vi "WebView2 Viewer.vi"(2 "ProjectRef":refnum<vi>, 4 "Extra Scripts":string, 5 "FileDependency In":map{path, T1}(c390), 6 "Options":string, 7 "OpenWebBrowser(False)":bool, 8 "error in":errorcluster, 9 "Embedd VISJS Librarya in HTMl File(False)":bool, 10 "HTMLFilePath":path, 11 "LibraryDependency":map{path, T3}(c390)) -> (0 "error out":errorcluster, 3 "HTMLFileContent":string)   [LabVIEW 2020, in "WebView2-Viewer.lvlib"] (continued)
if(d)e=g.iterator;else if(h)e=g;else{if(!(C=Wy(g)))throw new Uy(Gy(g)+\" is not iterable\");if(jy(C)){for(I=0,i=Ly(g);i>I;I++)if((o=p(g[I]))&&Vy(Ky,o))return o;return new _y(!1)}e=Yy(g,C)}for(n=d?g.next:e.next;!(r=Zy(n,e)).done;){try{o=p(r.value)}catch(g){Qy(e,\"throw\",g)}if(\"object\"==typeof o&&o&&Vy(Ky,o))return o}return new _y(!1)},Xy=og,Jy=TypeError,qy=function(g,t){if(Xy(t,g))return g;throw new Jy(\"Incorrect invocation\")},$y=TA,gm=C,tm=zy,Am=I,em=uA,Cm=Hy,Im=qy,im=O,om=gg,nm=Q,rm=_I,sm=Jt.f,am=Sr.forEach,dm=D,hm=GC.set,lm=GC.getterFor,cm=function(g,t,A){var e,C=-1!==g.indexOf(\"Map\"),I=-1!==g.indexOf(\"Weak\"),i=C?\"set\":\"add\",o=gm[g],n=o&&o.prototype,r={};if(dm&&im(o)&&(I||n.forEach&&!Am((function(){(new o).entries().next()})))){var s=(e=t((function(t,A){hm(Im(t,s),{type:g,collection:new o}),nm(A)||Cm(A,t[i],{that:t,AS_ENTRIES:C})}))).prototype,a=lm(g);am([\"add\",\"clear\",\"delete\",\"forEach\",\"get\",\"has\",\"set\",\"keys\",\"values\",\"entries\"],(function(g){var t=\"add\"===g||\"set\"===g;!(g in n)||I&&\"clear\"===g||em(s,g,(function(A,e){var C=a(this).collection;if(!t&&I&&!om(A))return\"get\"===g&&void 0;var i=C[g](0===A?0:A,e);return t?this:i}))})),I||sm(s,\"size\",{configurable:!0,get:function(){return a(this).collection.size}})}else e=A.getConstructor(t,g,C,i),tm.enable();return rm(e,g,!1,!0),r[g]=e,$y({global:!0,forced:!0},r),I||A.setStrong(e,g,C),e},um=TI,pm=function(g,t,A){for(var e in t)A&&A.unsafe&&g[e]?g[e]=t[e]:um(g,e,t[e],A);return g},fm=ig,vm=ur,ym=D,mm=dt(\"species\"),bm=function(g){var t=fm(g);ym&&t&&!t[mm]&&vm(t,mm,{configurable:!0,get:function(){return this}})},wm=pI,km=ur,xm=pm,Em=Xt,Om=qy,Tm=Q,Dm=Hy,Nm=Ei,Rm=Oi,Pm=bm,Mm=D,Bm=zy.fastKey,zm=GC.set,Sm=GC.getterFor,Zm={getConstructor:function(g,t,A,e){var C=g((function(g,C){Om(g,I),zm(g,{type:t,index:wm(null),first:void 0,last:void 0,size:0}),Mm||(g.size=0),Tm(C)||Dm(C,g[e],{that:g,AS_ENTRIES:A})})),I=C.prototype,i=Sm(t),o=function(g,t,A){var e,C,I=i(g),o=n(g,t);return o?o.value=A:(I.last=o={index:C=Bm(t,!0),key:t,value:A,previous:e=I.last,next:void 0,removed:!1},I.first||(I.first=o),e&&(e.next=o),Mm?I.size++:g.size++,\"F\"!==C&&(I.index[C]=o)),g},n=function(g,t){var A,e=i(g),C=Bm(t);if(\"F\"!==C)return e.index[C];for(A=e.first;A;A=A.next)if(A.key===t)return A};return xm(I,{clear:function(){for(var g=i(this),t=g.index,A=g.first;A;)A.removed=!0,A.previous&&(A.previous=A.previous.next=void 0),delete t[A.index],A=A.next;g.first=g.last=void 0,Mm?g.size=0:this.size=0},delete:function(g){var t=this,A=i(t),e=n(t,g);if(e){var C=e.next,I=e.previous;delete A.index[e.index],e.removed=!0,I&&(I.next=C),C&&(C.previous=I),A.first===e&&(A.first=C),A.last===e&&(A.last=I),Mm?A.size--:t.size--}return!!e},forEach:function(g){for(var t,A=i(this),e=Em(g,arguments.length>1?arguments[1]:void 0);t=t?t.next:A.first;)for(e(t.value,t.key,this);t&&t.removed;)t=t.previous},has:function(g){return!!n(this,g)}}),xm(I,A?{get:function(g){var t=n(this,g);return t&&t.value},set:function(g,t){return o(this,0===g?0:g,t)}}:{add:function(g){return o(this,g=0===g?0:g,g)}}),Mm&&km(I,\"size\",{configurable:!0,get:function(){return i(this).size}}),C},setStrong:function(g,t,A){var e=t+\" Iterator\",C=Sm(t),I=Sm(e);Nm(g,t,(function(g,t){zm(this,{type:e,target:g,state:C(g),kind:t,last:void 0})}),(function(){for(var g=I(this),t=g.kind,A=g.last;A&&A.removed;)A=A.previous;return g.target&&(g.last=A=A?A.next:g.state.first)?Rm(\"keys\"===t?A.key:\"values\"===t?A.value:[A.key,A.value],!1):(g.target=void 0,Rm(void 0,!0))}),A?\"entries\":\"values\",!A,!0),Pm(t)}};cm(\"Map\",(function(g){return function(){return g(this,arguments.length?arguments[0]:void 0)}}),Zm);var Fm=A(tg.Map),Gm=function(){function g(){cn(this,g),this.clear(),this._defaultIndex=0,this._groupIndex=0,this._defaultGroups=[{border:\"#2B7CE9\",background:\"#97C2FC\",highlight:{border:\"#2B7CE9\",background:\"#D2E5FF\"},hover:{border:\"#2B7CE9\",background:\"#D2E5FF\"}},{border:\"#FFA500\",background:\"#FFFF00\",highlight:{border:\"#FFA500\",background:\"#FFFFA3\"},hover:{border:\"#FFA500\",background:\"#FFFFA3\"}},{border:\"#FA0A10\",background:\"#FB7E81\",highlight:{border:\"#FA0A10\",background:\"#FFAFB1\"},hover:{border:\"#FA0A10\",background:\"#FFAFB1\"}},{border:\"#41A906\",background:\"#7BE141\",highlight:{border:\"#41A906\",background:\"#A1EC76\"},hover:{border:\"#41A906\",background:\"#A1EC76\"}},{border:\"#E129F0\",background:\"#EB7DF4\",highlight:{border:\"#E129F0\",background:\"#F0B3F5\"},hover:{border:\"#E129F0\",background:\"#F0B3F5\"}},{border:\"#7C29F0\",background:\"#AD85E4\",highlight:{border:\"#7C29F0\",background:\"#D3BDF0\"},hover:{border:\"#7C29F0\",background:\"#D3BDF0\"}},{border:\"#C37F00\",background:\"#FFA807\",highlight:{border:\"#C37F00\",background:\"#FFCA66\"},hover:{border:\"#C37F00\",background:\"#FFCA66\"}},{border:\"#4220FB\",background:\"#6E6EFD\",highlight:{border:\"#4220FB\",background:\"#9B9BFD\"},hover:{border:\"#4220FB\",background:\"#9B9BFD\"}},{border:\"#FD5A77\",background:\"#FFC0CB\",highlight:{border:\"#FD5A77\",background:\"#FFD1D9\"},hover:{border:\"#FD5A77\",background:\"#FFD1D9\"}},{border:\"#4AD63A\",background:\"#C2FABC\",highlight:{border:\"#4AD63A\",background:\"#E6FFE3\"},hover:{border:\"#4AD63A\",background:\"#E6FFE3\"}},{border:\"#990000\",background:\"#EE0000\",highlight:{border:\"#BB0000\",background:\"#FF3333\"},hover:{border:\"#BB0000\",background:\"#FF3333\"}},{border:\"#FF6000\",background:\"#FF6000\",highlight:{border:\"#FF6000\",background:\"#FF6000\"},hover:{border:\"#FF6000\",background:\"#FF6000\"}},{border:\"#97C2FC\",background:\"#2B7CE9\",highlight:{border:\"#D2E5FF\",background:\"#2B7CE9\"},hover:{border:\"#D2E5FF\",background:\"#2B7CE9\"}},{border:\"#399605\",background:\"#255C03\",highlight:{border:\"#399605\",background:\"#255C03\"},hover:{border:\"#399605\",background:\"#255C03\"}},{border:\"#B70054\",background:\"#FF007E\",highlight:{border:\"#B70054\",background:\"#FF007E\"},hover:{border:\"#B70054\",background:\"#FF007E\"}},{border:\"#AD85E4\",background:\"#7C29F0\",highlight:{border:\"#D3BDF0\",background:\"#7C29F0\"},hover:{border:\"#D3BDF0\",background:\"#7C29F0\"}},{border:\"#4557FA\",background:\"#000EA1\",highlight:{border:\"#6E6EFD\",background:\"#000EA1\"},hover:{border:\"#6E6EFD\",background:\"#000EA1\"}},{border:\"#FFC0CB\",background:\"#FD5A77\",highlight:{border:\"#FFD1D9\",background:\"#FD5A77\"},hover:{border:\"#FFD1D9\",background:\"#FD5A77\"}},{border:\"#C2FABC\",background:\"#74D66A\",highlight:{border:\"#E6FFE3\",background:\"#74D66A\"},hover:{border:\"#E6FFE3\",background:\"#74D66A\"}},{border:\"#EE0000\",background:\"#990000\",highlight:{border:\"#FF3333\",background:\"#BB0000\"},hover:{border:\"#FF3333\",background:\"#BB0000\"}}],this.options={},this.defaultOptions={useDefaultGroups:!0},fe(this.options,this.defaultOptions)}return kd(g,[{key:\"setOptions\",value:function(g){var t=[\"useDefaultGroups\"];if(void 0!==g)for(var A in g)if(Object.prototype.hasOwnProperty.call(g,A)&&-1===Xc(t).call(t,A)){var e=g[A];this.add(A,e)}}},{key:\"clear\",value:function(){this._groups=new Fm,this._groupNames=[]}},{key:\"get\",value:function(g){var t=!(arguments.length>1&&void 0!==arguments[1])||arguments[1],A=this._groups.get(g);if(void 0===A&&t)if(!1===this.options.useDefaultGroups&&this._groupNames.length>0){var e=this._groupIndex%this._groupNames.length;++this._groupIndex,(A={}).color=this._groups.get(this._groupNames[e]),this._groups.set(g,A)}else{var C=this._defaultIndex%this._defaultGroups.length;this._defaultIndex++,(A={}).color=this._defaultGroups[C],this._groups.set(g,A)}return A}},{key:\"add\",value:function(g,t){return this._groups.has(g)||this._groupNames.push(g),this._groups.set(g,t),t}}]),g}();TA({target:\"Number\",stat:!0},{isNaN:function(g){return g!=g}});var jm=A(tg.Number.isNaN),Lm=C.isFinite,Vm=Number.isFinite||function(g){return\"number\"==typeof g&&Lm(g)};TA({target:\"Number\",stat:!0},{isFinite:Vm});var Ym=A(tg.Number.isFinite),Wm=Sr.some;TA({target:\"Array\",proto:!0,forced:!_h(\"some\")},{some:function(g){return Wm(this,g,arguments.length>1?arguments[1]:void 0)}});var Qm=Me(\"Array\").some,Um=og,_m=Qm,Km=Array.prototype,Hm=function(g){var t=g.some;return g===Km||Um(Km,g)&&t===Km.some?_m:t},Xm=A(Hm);function Jm(g){if(void 0===g)throw new ReferenceError(\"this hasn't been initialised - super() hasn't been called\");return g}var qm=qc,$m=A(qm);TA({target:\"Object\",stat:!0},{setPrototypeOf:ri});var gb=tg.Object.setPrototypeOf,tb=A(gb),Ab=A(Ge);function eb(g,t){var A;return eb=tb?Ab(A=tb).call(A):function(g,t){return g.__proto__=t,g},eb(g,t)}function Cb(g,t){if(\"function\"!=typeof t&&null!==t)throw new TypeError(\"Super expression must either be null or a function\");g.prototype=$m(t&&t.prototype,{constructor:{value:g,writable:!0,configurable:!0}}),kn(g,\"prototype\",{writable:!1}),t&&eb(g,t)}function Ib(g,t){if(t&&(\"object\"===yd(t)||\"function\"==typeof t))return t;if(void 0!==t)throw new TypeError(\"Derived constructors may only return object or undefined\");return Jm(g)}var ib=rc,ob=A(ib);function nb(g){var t;return nb=tb?Ab(t=ob).call(t):function(g){return g.__proto__||ob(g)},nb(g)}function rb(g,t,A){return(t=bd(t))in g?kn(g,t,{value:A,enumerable:!0,configurable:!0,writable:!0}):g[t]=A,g}var sb={exports:{}},ab={exports:{}};!function(g){var t=cd,A=fd;function e(C){return g.exports=e=\"function\"==typeof t&&\"symbol\"==typeof A?function(g){return typeof g}:function(g){return g&&\"function\"==typeof t&&g.constructor===t&&g!==t.prototype?\"symbol\":typeof g},g.exports.__esModule=!0,g.exports.default=g.exports,e(C)}g.exports=e,g.exports.__esModule=!0,g.exports.default=g.exports}(ab);var db=ab.exports,hb=el,lb=qg,cb=Dh,ub=T,pb=Jt,fb=gg,vb=uA,yb=Error,mb=u(\"\".replace),bb=String(new yb(\"zxcasd\").stack),wb=/\\n\\s*at [^:]*:[^\\n]*/,kb=wb.test(bb),xb=G,Eb=!I((function(){var g=new Error(\"a\");return!(\"stack\"in g)||(Object.defineProperty(g,\"stack\",xb(1,7)),7!==g.stack)})),Ob=uA,Tb=function(g,t){if(kb&&\"string\"==typeof g&&!yb.prepareStackTrace)for(;t--;)g=mb(g,wb,\"\");return g},Db=Eb,Nb=Error.captureStackTrace,Rb=sC,Pb=TA,Mb=og,Bb=EI,zb=ri,Sb=function(g,t,A){for(var e=cb(t),C=pb.f,I=ub.f,i=0;i<e.length;i++){var o=e[i];lb(g,o)||A&&lb(A,o)||C(g,o,I(t,o))}},Zb=pI,Fb=uA,Gb=G,jb=function(g,t){fb(t)&&\"cause\"in t&&vb(g,\"cause\",t.cause)},Lb=function(g,t,A,e){Db&&(Nb?Nb(g,t):Ob(g,\"stack\",Tb(A,e)))},Vb=Hy,Yb=function(g,t){return void 0===g?arguments.length<2?\"\":t:Rb(g)},Wb=dt(\"toStringTag\"),Qb=Error,Ub=[].push,_b=function(g,t){var A,e=Mb(Kb,this);zb?A=zb(new Qb,e?Bb(this):Kb):(A=e?this:Zb(Kb),Fb(A,Wb,\"Error\")),void 0!==t&&Fb(A,\"message\",Yb(t)),Lb(A,_b,A.stack,1),arguments.length>2&&jb(A,arguments[2]);var C=[];return Vb(g,Ub,{that:C}),Fb(A,\"errors\",C),A};zb?zb(_b,Qb):Sb(_b,Qb,{name:!0});var Kb=_b.prototype=Zb(Qb.prototype,{constructor:Gb(1,_b),message:Gb(1,\"\"),name:Gb(1,\"AggregateError\")});Pb({global:!0,constructor:!0,arity:2},{AggregateError:_b});var Hb,Xb,Jb,qb,$b=\"process\"===y(C.process),gw=ro,tw=Og,Aw=TypeError,ew=function(g){if(gw(g))return g;throw new Aw(tw(g)+\" is not a constructor\")},Cw=AA,Iw=ew,iw=Q,ow=dt(\"species\"),nw=function(g,t){var A,e=Cw(g).constructor;return void 0===e||iw(A=Cw(e)[ow])?t:Iw(A)},rw=/(?:ipad|iphone|ipod).*applewebkit/i.test(ng),sw=C,aw=a,dw=Xt,hw=O,lw=qg,cw=I,uw=gI,pw=ve,fw=Et,vw=iu,yw=rw,mw=$b,bw=sw.setImmediate,ww=sw.clearImmediate,kw=sw.process,xw=sw.Dispatch,Ew=sw.Function,Ow=sw.MessageChannel,Tw=sw.String,Dw=0,Nw={},Rw=\"onreadystatechange\";cw((function(){Hb=sw.location}));var Pw=function(g){if(lw(Nw,g)){var t=Nw[g];delete Nw[g],t()}},Mw=function(g){return function(){Pw(g)}},Bw=function(g){Pw(g.data)},zw=function(g){sw.postMessage(Tw(g),Hb.protocol+\"//\"+Hb.host)};bw&&ww||(bw=function(g){vw(arguments.length,1);var t=hw(g)?g:Ew(g),A=pw(arguments,1);return Nw[++Dw]=function(){aw(t,void 0,A)},Xb(Dw),Dw},ww=function(g){delete Nw[g]},mw?Xb=function(g){kw.nextTick(Mw(g))}:xw&&xw.now?Xb=function(g){xw.now(Mw(g))}:Ow&&!yw?(qb=(Jb=new Ow).port2,Jb.port1.onmessage=Bw,Xb=dw(qb.postMessage,qb)):sw.addEventListener&&hw(sw.postMessage)&&!sw.importScripts&&Hb&&\"file:\"!==Hb.protocol&&!cw(zw)?(Xb=zw,sw.addEventListener(\"message\",Bw,!1)):Xb=Rw in fw(\"script\")?function(g){uw.appendChild(fw(\"script\"))[Rw]=function(){uw.removeChild(this),Pw(g)}}:function(g){setTimeout(Mw(g),0)});var Sw={set:bw,clear:ww},Zw=function(){this.head=null,this.tail=null};Zw.prototype={add:function(g){var t={item:g,next:null},A=this.tail;A?A.next=t:this.head=t,this.tail=t},get:function(){var g=this.head;if(g)return null===(this.head=g.next)&&(this.tail=null),g.item}};var Fw,Gw,jw,Lw,Vw,Yw=Zw,Ww=/ipad|iphone|ipod/i.test(ng)&&\"undefined\"!=typeof Pebble,Qw=/web0s(?!.*chrome)/i.test(ng),Uw=C,_w=Xt,Kw=T.f,Hw=Sw.set,Xw=Yw,Jw=rw,qw=Ww,$w=Qw,gk=$b,tk=Uw.MutationObserver||Uw.WebKitMutationObserver,Ak=Uw.document,ek=Uw.process,Ck=Uw.Promise,Ik=Kw(Uw,\"queueMicrotask\"),ik=Ik&&Ik.value;if(!ik){var ok=new Xw,nk=function(){var g,t;for(gk&&(g=ek.domain)&&g.exit();t=ok.get();)try{t()}catch(g){throw ok.head&&Fw(),g}g&&g.enter()};Jw||gk||$w||!tk||!Ak?!qw&&Ck&&Ck.resolve?((Lw=Ck.resolve(void 0)).constructor=Ck,Vw=_w(Lw.then,Lw),Fw=function(){Vw(nk)}):gk?Fw=function(){ek.nextTick(nk)}:(Hw=_w(Hw,Uw),Fw=function(){Hw(nk)}):(Gw=!0,jw=Ak.createTextNode(\"\"),new tk(nk).observe(jw,{characterData:!0}),Fw=function(){jw.data=Gw=!Gw}),ik=function(g){ok.head||Fw(),ok.add(g)}}var rk=ik,sk=function(g){try{return{error:!1,value:g()}}catch(g){return{error:!0,value:g}}},ak=C.Promise,dk=\"object\"==typeof Deno&&Deno&&\"object\"==typeof Deno.version,hk=!dk&&!$b&&\"object\"==typeof window&&\"object\"==typeof document,lk=C,ck=ak,uk=O,pk=Ut,fk=Hi,vk=dt,yk=hk,mk=dk,bk=cg,wk=ck&&ck.prototype,kk=vk(\"species\"),xk=!1,Ek=uk(lk.PromiseRejectionEvent),Ok=pk(\"Promise\",(function(){var g=fk(ck),t=g!==String(ck);if(!t&&66===bk)return!0;if(!wk.catch||!wk.finally)return!0;if(!bk||bk<51||!/native code/.test(g)){var A=new ck((function(g){g(1)})),e=function(g){g((function(){}),(function(){}))};if((A.constructor={})[kk]=e,!(xk=A.then((function(){}))instanceof e))return!0}return!t&&(yk||mk)&&!Ek})),Tk={CONSTRUCTOR:Ok,REJECTION_EVENT:Ek,SUBCLASSING:xk},Dk={},Nk=Rg,Rk=TypeError,Pk=function(g){var t,A;this.promise=new g((function(g,e){if(void 0!==t||void 0!==A)throw new Rk(\"Bad Promise constructor\");t=g,A=e})),this.resolve=Nk(t),this.reject=Nk(A)};Dk.f=function(g){return new Pk(g)};var Mk,Bk,zk=TA,Sk=$b,Zk=C,Fk=P,Gk=TI,jk=_I,Lk=bm,Vk=Rg,Yk=O,Wk=gg,Qk=qy,Uk=nw,_k=Sw.set,Kk=rk,Hk=function(g,t){try{1===arguments.length?console.error(g):console.error(g,t)}catch(g){}},Xk=sk,Jk=Yw,qk=GC,$k=ak,gx=Tk,tx=Dk,Ax=\"Promise\",ex=gx.CONSTRUCTOR,Cx=gx.REJECTION_EVENT,Ix=qk.getterFor(Ax),ix=qk.set,ox=$k&&$k.prototype,nx=$k,rx=ox,sx=Zk.TypeError,ax=Zk.document,dx=Zk.process,hx=tx.f,lx=hx,cx=!!(ax&&ax.createEvent&&Zk.dispatchEvent),ux=\"unhandledrejection\",px=function(g){var t;return!(!Wk(g)||!Yk(t=g.then))&&t},fx=function(g,t){var A,e,C,I=t.value,i=1===t.state,o=i?g.ok:g.fail,n=g.resolve,r=g.reject,s=g.domain;try{o?(i||(2===t.rejection&&wx(t),t.rejection=1),!0===o?A=I:(s&&s.enter(),A=o(I),s&&(s.exit(),C=!0)),A===g.promise?r(new sx(\"Promise-chain cycle\")):(e=px(A))?Fk(e,A,n,r):n(A)):r(I)}catch(g){s&&!C&&s.exit(),r(g)}},vx=function(g,t){g.notified||(g.notified=!0,Kk((function(){for(var A,e=g.reactions;A=e.get();)fx(A,g);g.notified=!1,t&&!g.rejection&&mx(g)})))},yx=function(g,t,A){var e,C;cx?((e=ax.createEvent(\"Event\")).promise=t,e.reason=A,e.initEvent(g,!1,!0),Zk.dispatchEvent(e)):e={promise:t,reason:A},!Cx&&(C=Zk[\"on\"+g])?C(e):g===ux&&Hk(\"Unhandled promise rejection\",A)},mx=function(g){Fk(_k,Zk,(function(){var t,A=g.facade,e=g.value;if(bx(g)&&(t=Xk((function(){Sk?dx.emit(\"unhandledRejection\",e,A):yx(ux,A,e)})),g.rejection=Sk||bx(g)?2:1,t.error))throw t.value}))},bx=function(g){return 1!==g.rejection&&!g.parent},wx=function(g){Fk(_k,Zk,(function(){var t=g.facade;Sk?dx.emit(\"rejectionHandled\",t):yx(\"rejectionhandled\",t,g.value)}))},kx=function(g,t,A){return function(e){g(t,e,A)}},xx=function(g,t,A){g.done||(g.done=!0,A&&(g=A),g.value=t,g.state=2,vx(g,!0))},Ex=function(g,t,A){if(!g.done){g.done=!0,A&&(g=A);try{if(g.facade===t)throw new sx(\"Promise can't be resolved itself\");var e=px(t);e?Kk((function(){var A={done:!1};try{Fk(e,t,kx(Ex,A,g),kx(xx,A,g))}catch(t){xx(A,t,g)}})):(g.value=t,g.state=1,vx(g,!1))}catch(t){xx({done:!1},t,g)}}};ex&&(rx=(nx=function(g){Qk(this,rx),Vk(g),Fk(Mk,this);var t=Ix(this);try{g(kx(Ex,t),kx(xx,t))}catch(g){xx(t,g)}}).prototype,(Mk=function(g){ix(this,{type:Ax,done:!1,notified:!1,parent:!1,reactions:new Jk,rejection:!1,state:0,value:void 0})}).prototype=Gk(rx,\"then\",(function(g,t){var A=Ix(this),e=hx(Uk(this,nx));return A.parent=!0,e.ok=!Yk(g)||g,e.fail=Yk(t)&&t,e.domain=Sk?dx.domain:void 0,0===A.state?A.reactions.add(e):Kk((function(){fx(e,A)})),e.promise})),Bk=function(){var g=new Mk,t=Ix(g);this.promise=g,this.resolve=kx(Ex,t),this.reject=kx(xx,t)},tx.f=hx=function(g){return g===nx||undefined===g?new Bk(g):lx(g)}),zk({global:!0,constructor:!0,wrap:!0,forced:ex},{Promise:nx}),jk(nx,Ax,!1,!0),Lk(Ax);var Ox=ak,Tx=Tk.CONSTRUCTOR||!Yo((function(g){Ox.all(g).then(void 0,(function(){}))})),Dx=P,Nx=Rg,Rx=Dk,Px=sk,Mx=Hy;TA({target:\"Promise\",stat:!0,forced:Tx},{all:function(g){var t=this,A=Rx.f(t),e=A.resolve,C=A.reject,I=Px((function(){var A=Nx(t.resolve),I=[],i=0,o=1;Mx(g,(function(g){var n=i++,r=!1;o++,Dx(A,t,g).then((function(g){r||(r=!0,I[n]=g,--o||e(I))}),C)})),--o||e(I)}));return I.error&&C(I.value),A.promise}});var Bx=TA,zx=Tk.CONSTRUCTOR;ak&&ak.prototype,Bx({target:\"Promise\",proto:!0,forced:zx,real:!0},{catch:function(g){return this.then(void 0,g)}});var Sx=P,Zx=Rg,Fx=Dk,Gx=sk,jx=Hy;TA({target:\"Promise\",stat:!0,forced:Tx},{race:function(g){var t=this,A=Fx.f(t),e=A.reject,C=Gx((function(){var C=Zx(t.resolve);jx(g,(function(g){Sx(C,t,g).then(A.resolve,e)}))}));return C.error&&e(C.value),A.promise}});var Lx=P,Vx=Dk;TA({target:\"Promise\",stat:!0,forced:Tk.CONSTRUCTOR},{reject:function(g){var t=Vx.f(this);return Lx(t.reject,void 0,g),t.promise}});var Yx=AA,Wx=gg,Qx=Dk,Ux=function(g,t){if(Yx(g),Wx(t)&&t.constructor===g)return t;var A=Qx.f(g);return(0,A.resolve)(t),A.promise},_x=TA,Kx=ak,Hx=Tk.CONSTRUCTOR,Xx=Ux,Jx=ig(\"Promise\"),qx=!Hx;_x({target:\"Promise\",stat:!0,forced:true},{resolve:function(g){return Xx(qx&&this===Jx?Kx:this,g)}});var $x=P,gE=Rg,tE=Dk,AE=sk,eE=Hy;TA({target:\"Promise\",stat:!0,forced:Tx},{allSettled:function(g){var t=this,A=tE.f(t),e=A.resolve,C=A.reject,I=AE((function(){var A=gE(t.resolve),C=[],I=0,i=1;eE(g,(function(g){var o=I++,n=!1;i++,$x(A,t,g).then((function(g){n||(n=!0,C[o]={status:\"fulfilled\",value:g},--i||e(C))}),(function(g){n||(n=!0,C[o]={status:\"rejected\",reason:g},--i||e(C))}))})),--i||e(C)}));return I.error&&C(I.value),A.promise}});var CE=P,IE=Rg,iE=ig,oE=Dk,nE=sk,rE=Hy,sE=\"No one promise resolved\";TA({target:\"Promise\",stat:!0,forced:Tx},{any:function(g){var t=this,A=iE(\"AggregateError\"),e=oE.f(t),C=e.resolve,I=e.reject,i=nE((function(){var e=IE(t.resolve),i=[],o=0,n=1,r=!1;rE(g,(function(g){var s=o++,a=!1;n++,CE(e,t,g).then((function(g){a||r||(r=!0,C(g))}),(function(g){a||r||(a=!0,i[s]=g,--n||I(new A(i,sE)))}))})),--n||I(new A(i,sE))}));return i.error&&I(i.value),e.promise}});var aE=TA,dE=ak,hE=I,lE=ig,cE=O,uE=nw,pE=Ux,fE=dE&&dE.prototype;aE({target:\"Promise\",proto:!0,real:!0,forced:!!dE&&hE((function(){fE.finally.call({then:function(){}},(function(){}))}))},{finally:function(g){var t=uE(this,lE(\"Promise\")),A=cE(g);return this.then(A?function(A){return pE(t,g()).then((function(){return A}))}:g,A?function(A){return pE(t,g()).then((function(){throw A}))}:g)}});var vE=tg.Promise,yE=Dk;TA({target:\"Promise\",stat:!0},{withResolvers:function(){var g=yE.f(this);return{promise:g.promise,resolve:g.resolve,reject:g.reject}}});var mE=vE,bE=Dk,wE=sk;TA({target:\"Promise\",stat:!0,forced:!0},{try:function(g){var t=bE.f(this),A=wE(g);return(A.error?t.reject:t.resolve)(A.value),
